vi "CaseStructure-Ver1-RadioButtons.vi"() -> ()   [LabVIEW 2018]
panel:
  in  "?":bool
  out "Radio Button Selection":string
  in  "Radio Buttons":enum32{"Option 1", "Option 2", "Option 3"}(radio)
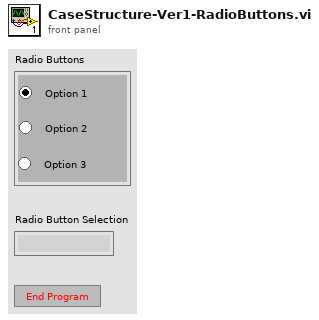
[diagram p1: front panel]
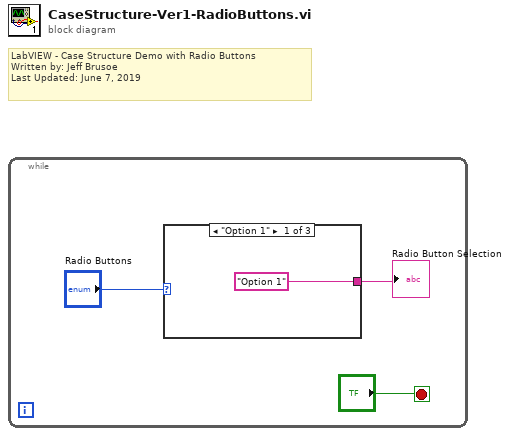
[diagram p0: block diagram]
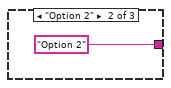
[diagram p2: hidden frame]
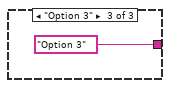
[diagram p3: hidden frame]
diagram:
  # "LabVIEW - Case Structure Demo with Radio Buttons\nWritten by: Jeff Brusoe\nLast Updated: June 7, 2019"
  n1 = while {
    stop <- "?" stop-if-true
    n2 = case shown="\"Option 1\"" "Radio Buttons" {
      tunnel: ["Option 1" "Option 2" "Option 3"] -> w2
      frame "Option 1" {
      }
      frame "Option 2" {
      }
      frame "Option 3" {
      }
    }
    "Radio Button Selection" <- w2
  }
